vi "Init Module.vi"(7 "Create from class input? (F)":bool, 8 "error in (no error)":errorcluster, 9 "RSI Module in":refnum<class "RSI Module.lvclass">, 10 "Slot Settings":T1, 11 "Module Model":T2) -> (0 "error out":errorcluster, 3 "RSI Module out":refnum<class "RSI Module.lvclass">)   [LabVIEW 2017, in "Modules.lvlib"]
uses:
  Modules.lvlib
  RSI Module/Module Models.ctl
  RSI Module/Slot Settings.ctl
  RSI Module/RSI Module.lvclass
  RSI Module/Channels.ctl
  RSI Module/Channel Type.ctl
  9213/9213.lvclass
  C:/Users/nitest/Documents/niveristand-scan-engine-module-libraries/Source/RSI Module/RSI Module.lvclass
  9203/9203.lvclass
  9205/9205.lvclass
  9207/9207.lvclass
  9211/9211.lvclass
  9212/9212.lvclass
  9214/9214.lvclass
  9217/9217.lvclass
  9219/9219.lvclass
  9229/9229.lvclass
  9233/9233.lvclass
  9234/9234.lvclass
  9235/9235.lvclass
  9237/9237.lvclass
  9239/9239.lvclass
  9242/9242.lvclass
  9244/9244.lvclass
  9401/9401.lvclass
  9402/9402.lvclass
  9403/9403.lvclass
  9478/9478.lvclass
  SD Module/SD Module.lvclass
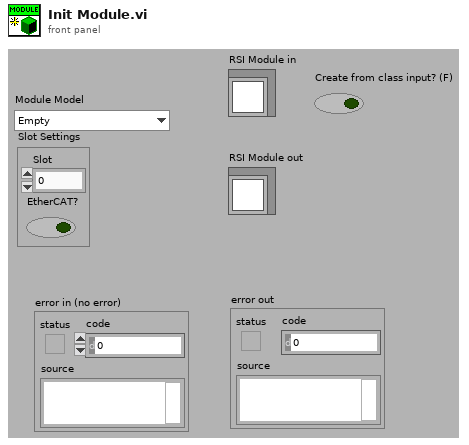
[diagram p1: front panel]
types:
  T1 = typedef "Modules.lvlib/RSI Module.lvclass/Slot Settings.ctl" = cluster{"Slot":u32, "EtherCAT?":bool}
  T2 = typedef "Modules.lvlib/RSI Module.lvclass/Module Models.ctl" = enum16{"Empty", "NI 9201", "NI 9203", "NI 9205", "NI 9206", "NI 9207", "NI 9208", "NI 9211", "NI 9212", "NI 9213", "NI 9214", "NI 9215", "NI 9217", "NI 9219", "NI 9220", "NI 9221", "NI 9222", "NI 9223", "NI 9224", "NI 9225", "NI 9227", "NI 9229", "NI 9233", "NI 9234", "NI 9235", "NI 9236", "NI 9237", "NI 9239", "NI 9242", "NI 9244", "NI 9263", "NI 9264", "NI 9265", "NI 9266", "NI 9269", "NI 9375", "NI 9401", "NI 9402", "NI 9403", "NI 9411", "NI 9421", "NI 9422", "NI 9423", "NI 9425", "NI 9426", "NI 9435", "NI 9437", "NI 9472", "NI 9474", "NI 9475", "NI 9476", "NI 9477", "NI 9478", "NI 9481", "NI 9482", "NI 9485"}
  T3 = typedef "Modules.lvlib/RSI Module.lvclass/Channels.ctl" = cluster{"# Input Channels":i32, "# Output Channels":i32, "Channel Type":T4, "Units":string}
  T4 = typedef "Modules.lvlib/RSI Module.lvclass/Channel Type.ctl" = enum16{"Analog", "Digital"}
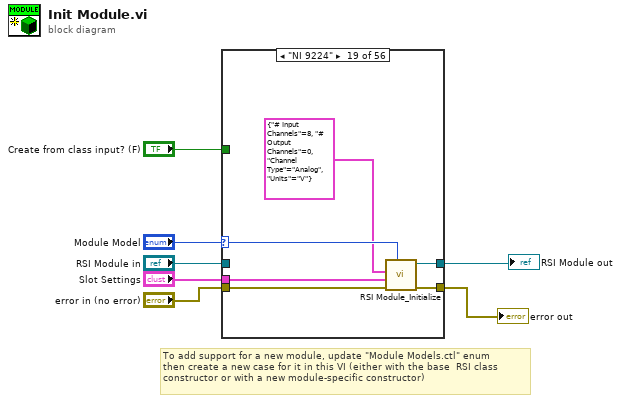
[diagram p0: block diagram]
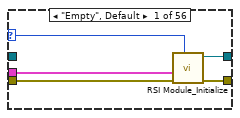
[diagram p2: hidden frame]
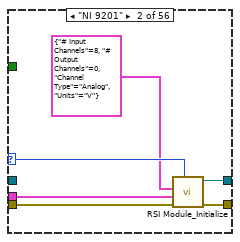
[diagram p3: hidden frame]
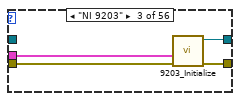
[diagram p4: hidden frame]
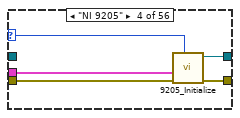
[diagram p5: hidden frame]
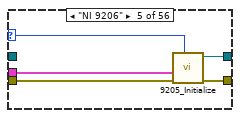
[diagram p6: hidden frame]
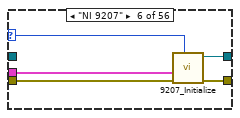
[diagram p7: hidden frame]
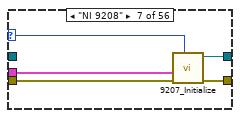
[diagram p8: hidden frame]
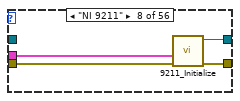
[diagram p9: hidden frame]
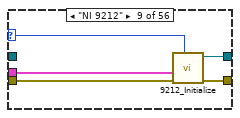
[diagram p10: hidden frame]
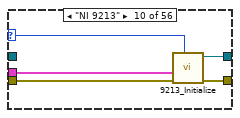
[diagram p11: hidden frame]
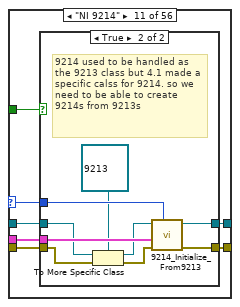
[diagram p12: hidden frame]
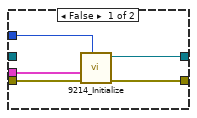
[diagram p13: hidden frame]
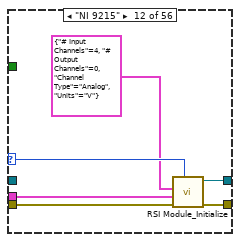
[diagram p14: hidden frame]
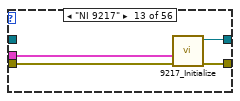
[diagram p15: hidden frame]
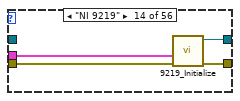
[diagram p16: hidden frame]
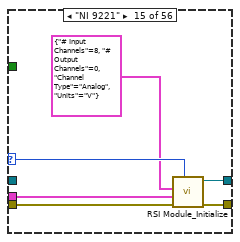
[diagram p17: hidden frame]
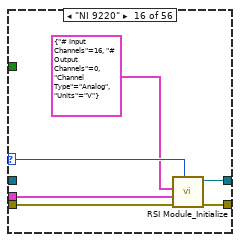
[diagram p18: hidden frame]
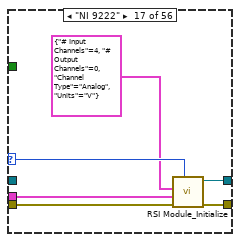
[diagram p19: hidden frame]
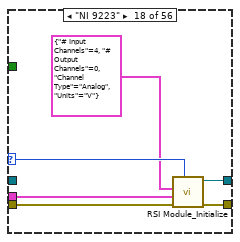
[diagram p20: hidden frame]
diagram:
  # "To add support for a new module, update \"Module Models.ctl\" enum\nthen create a new case for it in this VI (either with the base  RSI class\nconstructor or with a new module-specific constructor)"
  n1 = case shown="\"NI 9224\"" "Module Model" {
    selector: "Module Model" -> [w8 w18 _ w23 w29 w33 w38 _ w47 w52 w59 w83 _ _ w97 w103 w109 w115 w121 w127 w133 _ _ _ w146 w151 _ _ _ _ w177 w183 w189 w195 w201 w207 _ _ _ w226 w242 w260 w280 w301 w307 w310 w330 w348 w365 w386 w408 w414 _ w424 w430 w436]
    tunnel: [w11 w17 w19 w25 w31 w35 w40 w44 w50 w55 w62 w82 w87 w91 w96 w102 w108 w114 w120 w126 w132 w136 w140 w145 w150 w155 w157 w162 w164 w168 w176 w182 w188 w194 w200 w206 w211 w215 w219 w225 w244 w262 w282 w300 w306 w313 w332 w351 w370 w389 w407 w413 w417 w423 w429 w435] -> w3
    tunnel: [w12 w16 w22 w26 w32 w36 w41 w45 w51 w56 w63 w81 w86 w90 w95 w101 w107 w113 w119 w125 w131 w137 w141 w144 w147 w152 w156 w163 w167 w171 w175 w181 w187 w193 w199 w205 w210 w214 w218 w224 w243 w263 w277 w299 w305 w312 w331 w350 w369 w388 w406 w412 w418 w422 w428 w434] -> w6
    tunnel: "Slot Settings" -> [w9 w14 w20 w27 w28 w37 w42 w46 w48 w53 w60 w79 w85 w89 w93 w99 w105 w111 w117 w123 w129 w134 w139 w143 w148 w153 w158 w160 w165 w169 w173 w179 w185 w191 w197 w203 w209 w213 w217 w221 w240 w259 w279 w297 w303 w309 w328 w346 w367 w384 w404 w410 w415 w420 w426 w432]
    tunnel: "error in (no error)" -> [w10 w13 w21 w24 w30 w34 w39 w43 w49 w54 w61 w78 w84 w88 w92 w98 w104 w110 w116 w122 w128 w135 w138 w142 w149 w154 w159 w161 w166 w170 w172 w178 w184 w190 w196 w202 w208 w212 w216 w222 w241 w258 w278 w296 w302 w308 w329 w347 w368 w385 w403 w409 w416 w419 w425 w431]
    tunnel: "Create from class input? (F)" -> [_ _ _ _ _ _ _ _ _ _ w58 _ _ _ _ _ _ _ _ _ _ _ _ _ _ _ _ _ _ _ _ _ _ _ _ _ _ _ _ _ _ _ _ _ _ _ _ _ _ _ _ _ _ _ _ _]
    tunnel: "RSI Module in" -> [_ _ _ _ _ _ _ _ _ _ w57 _ _ _ _ _ _ _ _ _ _ _ _ _ _ _ _ _ _ _ _ _ _ _ _ _ _ _ _ _ _ _ _ _ _ _ _ _ _ _ _ _ _ _ _ _]
    frame "Empty", Default {
      n2 = call "RSI Module_Initialize.vi"("Module Model"=w8, "error in (no error)"=w10, "Slot Settings"=w9) -> ("error out"=w12:errorcluster, "RSI Module out"=w11:refnum<class "RSI Module.lvclass">)  [unwired: 7 in]
    }
    frame "NI 9201" {
      n3 = call "RSI Module_Initialize.vi"("Module Model"=w18, "error in (no error)"=w13, "Slot Settings"=w14, "Channels"=T3 {"# Input Channels"=8, "# Output Channels"=0, "Channel Type"=enum."Analog", "Units"="V"}) -> ("error out"=w16:errorcluster, "RSI Module out"=w17:refnum<class "RSI Module.lvclass">)  [unwired: 6 in]
    }
    frame "NI 9203" {
      n4 = call "9203_Initialize.vi"("error in (no error)"=w21, "Slot Settings"=w20) -> ("error out"=w22:errorcluster, "9203 out"=w19:refnum<class "9203.lvclass">)  [unwired: 8 in]
    }
    frame "NI 9205" {
      n5 = call "9205_Initialize.vi"("Module Model"=w23, "error in (no error)"=w24, "Slot Settings"=w27) -> ("error out"=w26:errorcluster, "9205 out"=w25:refnum<class "9205.lvclass">)  [unwired: 7 in]
    }
    frame "NI 9206" {
      n6 = call "9205_Initialize.vi"("Module Model"=w29, "error in (no error)"=w30, "Slot Settings"=w28) -> ("error out"=w32:errorcluster, "9205 out"=w31:refnum<class "9205.lvclass">)  [unwired: 7 in]
    }
    frame "NI 9207" {
      n7 = call "9207_Initialize.vi"("Module Model"=w33, "error in (no error)"=w34, "Slot Settings"=w37) -> ("error out"=w36:errorcluster, "9207 out"=w35:refnum<class "9207.lvclass">)  [unwired: 7 in]
    }
    frame "NI 9208" {
      n8 = call "9207_Initialize.vi"("Module Model"=w38, "error in (no error)"=w39, "Slot Settings"=w42) -> ("error out"=w41:errorcluster, "9207 out"=w40:refnum<class "9207.lvclass">)  [unwired: 7 in]
    }
    frame "NI 9211" {
      n9 = call "9211_Initialize.vi"("error in (no error)"=w43, "Slot Settings"=w46) -> ("error out"=w45:errorcluster, "9211 out"=w44:refnum<class "9211.lvclass">)  [unwired: 8 in]
    }
    frame "NI 9212" {
      n10 = call "9212_Initialize.vi"("Module Model"=w47, "error in (no error)"=w49, "Slot Settings"=w48) -> ("error out"=w51:errorcluster, "9213 out"=w50:refnum<class "9212.lvclass">)  [unwired: 7 in]
    }
    frame "NI 9213" {
      n11 = call "9213_Initialize.vi"("Module Model"=w52, "error in (no error)"=w54, "Slot Settings"=w53) -> ("error out"=w56:errorcluster, "9213 out"=w55:refnum<class "9213.lvclass">)  [unwired: 7 in]
    }
    frame "NI 9214" {
      n12 = case shown="True" w58 {
        tunnel: [w68 w77] -> w63
        tunnel: [w67 w76] -> w62
        tunnel: w61 -> [w66 w73]
        tunnel: w60 -> [w65 w75]
        tunnel: w59 -> [w64 w74]
        tunnel: w57 -> [_ w72]
        frame False {
          n13 = call "9214_Initialize.vi"("Module Model"=w64, "error in (no error)"=w66, "Slot Settings"=w65) -> ("error out"=w68:errorcluster, "9214 out"=w67:refnum<class "9214.lvclass">)  [unwired: 7 in]
        }
        frame True {
          # "9214 used to be handled as the 9213 class but 4.1 made a specific calss for 9214. so we need to be able to create 9214s from 9213s"
          n14 = To More Specific Class(target class=refnum<class "9213.lvclass"> refnum ("Modules.lvlib:9213.lvclass"), reference=w72, error in=w73) -> (specific class reference=w70:refnum<class "9213.lvclass">, error out=w69:errorcluster)
          n15 = call "9214_Initialize_From9213.vi"("Module Model"=w74, "error in (no error)"=w69, "Slot Settings"=w75, "9213 in"=w70) -> ("error out"=w77:errorcluster, "9214 out"=w76:refnum<class "9214.lvclass">)  [unwired: 6 in]
        }
      }
    }
    frame "NI 9215" {
      n16 = call "RSI Module_Initialize.vi"("Module Model"=w83, "error in (no error)"=w78, "Slot Settings"=w79, "Channels"=T3 {"# Input Channels"=4, "# Output Channels"=0, "Channel Type"=enum."Analog", "Units"="V"}) -> ("error out"=w81:errorcluster, "RSI Module out"=w82:refnum<class "RSI Module.lvclass">)  [unwired: 6 in]
    }
    frame "NI 9217" {
      n17 = call "9217_Initialize.vi"("error in (no error)"=w84, "Slot Settings"=w85) -> ("error out"=w86:errorcluster, "9217 out"=w87:refnum<class "9217.lvclass">)  [unwired: 8 in]
    }
    frame "NI 9219" {
      n18 = call "9219_Initialize.vi"("error in (no error)"=w88, "Slot Settings"=w89) -> ("error out"=w90:errorcluster, "9219 out"=w91:refnum<class "9219.lvclass">)  [unwired: 8 in]
    }
    frame "NI 9221" {
      n19 = call "RSI Module_Initialize.vi"("Module Model"=w97, "error in (no error)"=w92, "Slot Settings"=w93, "Channels"=T3 {"# Input Channels"=8, "# Output Channels"=0, "Channel Type"=enum."Analog", "Units"="V"}) -> ("error out"=w95:errorcluster, "RSI Module out"=w96:refnum<class "RSI Module.lvclass">)  [unwired: 6 in]
    }
    frame "NI 9220" {
      n20 = call "RSI Module_Initialize.vi"("Module Model"=w103, "error in (no error)"=w98, "Slot Settings"=w99, "Channels"=T3 {"# Input Channels"=16, "# Output Channels"=0, "Channel Type"=enum."Analog", "Units"="V"}) -> ("error out"=w101:errorcluster, "RSI Module out"=w102:refnum<class "RSI Module.lvclass">)  [unwired: 6 in]
    }
    frame "NI 9222" {
      n21 = call "RSI Module_Initialize.vi"("Module Model"=w109, "error in (no error)"=w104, "Slot Settings"=w105, "Channels"=T3 {"# Input Channels"=4, "# Output Channels"=0, "Channel Type"=enum."Analog", "Units"="V"}) -> ("error out"=w107:errorcluster, "RSI Module out"=w108:refnum<class "RSI Module.lvclass">)  [unwired: 6 in]
    }
    frame "NI 9223" {
      n22 = call "RSI Module_Initialize.vi"("Module Model"=w115, "error in (no error)"=w110, "Slot Settings"=w111, "Channels"=T3 {"# Input Channels"=4, "# Output Channels"=0, "Channel Type"=enum."Analog", "Units"="V"}) -> ("error out"=w113:errorcluster, "RSI Module out"=w114:refnum<class "RSI Module.lvclass">)  [unwired: 6 in]
    }
    frame "NI 9224" {
      n23 = call "RSI Module_Initialize.vi"("Module Model"=w121, "error in (no error)"=w116, "Slot Settings"=w117, "Channels"=T3 {"# Input Channels"=8, "# Output Channels"=0, "Channel Type"=enum."Analog", "Units"="V"}) -> ("error out"=w119:errorcluster, "RSI Module out"=w120:refnum<class "RSI Module.lvclass">)  [unwired: 6 in]
    }
    frame "NI 9225" {
      n24 = call "RSI Module_Initialize.vi"("Module Model"=w127, "error in (no error)"=w122, "Slot Settings"=w123, "Channels"=T3 {"# Input Channels"=3, "# Output Channels"=0, "Channel Type"=enum."Analog", "Units"="Vrms"}) -> ("error out"=w125:errorcluster, "RSI Module out"=w126:refnum<class "RSI Module.lvclass">)  [unwired: 6 in]
    }
    frame "NI 9227" {
      n25 = call "RSI Module_Initialize.vi"("Module Model"=w133, "error in (no error)"=w128, "Slot Settings"=w129, "Channels"=T3 {"# Input Channels"=4, "# Output Channels"=0, "Channel Type"=enum."Analog", "Units"="Arms"}) -> ("error out"=w131:errorcluster, "RSI Module out"=w132:refnum<class "RSI Module.lvclass">)  [unwired: 6 in]
    }
    frame "NI 9229" {
      n26 = call "9229_Initialize.vi"("error in (no error)"=w135, "Slot Settings"=w134) -> ("error out"=w137:errorcluster, "9229 out"=w136:refnum<class "9229.lvclass">)  [unwired: 8 in]
    }
    frame "NI 9233" {
      n27 = call "9233_Initialize.vi"("error in (no error)"=w138, "Slot Settings"=w139) -> ("error out"=w141:errorcluster, "9233 out"=w140:refnum<class "9233.lvclass">)  [unwired: 8 in]
    }
    frame "NI 9234" {
      n28 = call "9234_Initialize.vi"("error in (no error)"=w142, "Slot Settings"=w143) -> ("error out"=w144:errorcluster, "9234 out"=w145:refnum<class "9234.lvclass">)  [unwired: 8 in]
    }
    frame "NI 9235" {
      n29 = call "9235_Initialize.vi"("Module Model"=w146, "error in (no error)"=w149, "Slot Settings"=w148) -> ("error out"=w147:errorcluster, "9235 out"=w150:refnum<class "9235.lvclass">)  [unwired: 7 in]
    }
    frame "NI 9236" {
      n30 = call "9235_Initialize.vi"("Module Model"=w151, "error in (no error)"=w154, "Slot Settings"=w153) -> ("error out"=w152:errorcluster, "9235 out"=w155:refnum<class "9235.lvclass">)  [unwired: 7 in]
    }
    frame "NI 9237" {
      n31 = call "9237_Initialize.vi"("error in (no error)"=w159, "Slot Settings"=w158) -> ("error out"=w156:errorcluster, "9237 out"=w157:refnum<class "9237.lvclass">)  [unwired: 8 in]
    }
    frame "NI 9239" {
      n32 = call "9239_Initialize.vi"("error in (no error)"=w161, "Slot Settings"=w160) -> ("error out"=w163:errorcluster, "9239 out"=w162:refnum<class "9239.lvclass">)  [unwired: 8 in]
    }
    frame "NI 9242" {
      n33 = call "9242_Initialize.vi"("error in (no error)"=w166, "Slot Settings"=w165) -> ("error out"=w167:errorcluster, "Modules.lvlib:9242.lvclass"=w164:refnum<class "9242.lvclass">)  [unwired: 8 in]
    }
    frame "NI 9244" {
      n34 = call "9244_Initialize.vi"("error in (no error)"=w170, "Slot Settings"=w169) -> ("error out"=w171:errorcluster, "Modules.lvlib:9244.lvclass"=w168:refnum<class "9244.lvclass">)  [unwired: 8 in]
    }
    frame "NI 9263" {
      n35 = call "RSI Module_Initialize.vi"("Module Model"=w177, "error in (no error)"=w172, "Slot Settings"=w173, "Channels"=T3 {"# Input Channels"=0, "# Output Channels"=4, "Channel Type"=enum."Analog", "Units"="V"}) -> ("error out"=w175:errorcluster, "RSI Module out"=w176:refnum<class "RSI Module.lvclass">)  [unwired: 6 in]
    }
    frame "NI 9264" {
      n36 = call "RSI Module_Initialize.vi"("Module Model"=w183, "error in (no error)"=w178, "Slot Settings"=w179, "Channels"=T3 {"# Input Channels"=0, "# Output Channels"=16, "Channel Type"=enum."Analog", "Units"="V"}) -> ("error out"=w181:errorcluster, "RSI Module out"=w182:refnum<class "RSI Module.lvclass">)  [unwired: 6 in]
    }
    frame "NI 9265" {
      n37 = call "RSI Module_Initialize.vi"("Module Model"=w189, "error in (no error)"=w184, "Slot Settings"=w185, "Channels"=T3 {"# Input Channels"=0, "# Output Channels"=4, "Channel Type"=enum."Analog", "Units"="A"}) -> ("error out"=w187:errorcluster, "RSI Module out"=w188:refnum<class "RSI Module.lvclass">)  [unwired: 6 in]
    }
    frame "NI 9266" {
      n38 = call "RSI Module_Initialize.vi"("Module Model"=w195, "error in (no error)"=w190, "Slot Settings"=w191, "Channels"=T3 {"# Input Channels"=0, "# Output Channels"=8, "Channel Type"=enum."Analog", "Units"="A"}) -> ("error out"=w193:errorcluster, "RSI Module out"=w194:refnum<class "RSI Module.lvclass">)  [unwired: 6 in]
    }
    frame "NI 9269" {
      n39 = call "RSI Module_Initialize.vi"("Module Model"=w201, "error in (no error)"=w196, "Slot Settings"=w197, "Channels"=T3 {"# Input Channels"=0, "# Output Channels"=4, "Channel Type"=enum."Analog", "Units"="V"}) -> ("error out"=w199:errorcluster, "RSI Module out"=w200:refnum<class "RSI Module.lvclass">)  [unwired: 6 in]
    }
    frame "NI 9375" {
      n40 = call "RSI Module_Initialize.vi"("Module Model"=w207, "error in (no error)"=w202, "Slot Settings"=w203, "Channels"=T3 {"# Input Channels"=16, "# Output Channels"=16, "Channel Type"=enum."Digital", "Units"=""}) -> ("error out"=w205:errorcluster, "RSI Module out"=w206:refnum<class "RSI Module.lvclass">)  [unwired: 6 in]
    }
    frame "NI 9401" {
      n41 = call "9401_Initialize.vi"("error in (no error)"=w208, "Slot Settings"=w209) -> ("error out"=w210:errorcluster, "9401 out"=w211:refnum<class "9401.lvclass">)  [unwired: 8 in]
    }
    frame "NI 9402" {
      n42 = call "9402_Initialize.vi"("error in (no error)"=w212, "Slot Settings"=w213) -> ("error out"=w214:errorcluster, "9402 out"=w215:refnum<class "9402.lvclass">)  [unwired: 8 in]
    }
    frame "NI 9403" {
      n43 = call "9403_Initialize.vi"("error in (no error)"=w216, "Slot Settings"=w217) -> ("error out"=w218:errorcluster, "9403 out"=w219:refnum<class "9403.lvclass">)  [unwired: 8 in]
    }
    frame "NI 9411" {
      n44 = Unbundle By Name(w221) -> ("EtherCAT?"=w220:bool)
      n45 = case shown="True" w220 {
        tunnel: w226 -> [w232 w235]
        tunnel: [w231 w236] -> w225
        tunnel: [w230 w237] -> w224
        tunnel: T3 {"# Input Channels"=6, "# Output Channels"=0, "Channel Type"=enum."Digital", "Units"=""} ("Channels") -> [w229 w234]
        tunnel: w222 -> [w228 w238]
        tunnel: w221 -> [w227 w233]
        frame False {
          n46 = call "SD Module_Initialize.vi"("Module Model"=w232, "error in (no error)"=w228, "Slot Settings"=w227, "Channels"=w229) -> ("error out"=w230:errorcluster, "SD Module out"=w231:refnum<class "SD Module.lvclass">)  [unwired: 6 in]
        }
        frame True {
          n47 = call "RSI Module_Initialize.vi"("Module Model"=w235, "error in (no error)"=w238, "Slot Settings"=w233, "Channels"=w234) -> ("error out"=w237:errorcluster, "RSI Module out"=w236:refnum<class "RSI Module.lvclass">)  [unwired: 6 in]
        }
      }
    }
    frame "NI 9421" {
      n48 = Unbundle By Name(w240) -> ("EtherCAT?"=w245:bool)
      n49 = case shown="True" w245 {
        tunnel: w242 -> [w251 w254]
        tunnel: [w250 w255] -> w244
        tunnel: [w249 w256] -> w243
        tunnel: T3 {"# Input Channels"=8, "# Output Channels"=0, "Channel Type"=enum."Digital", "Units"=""} ("Channels") -> [w248 w253]
        tunnel: w241 -> [w247 w257]
        tunnel: w240 -> [w246 w252]
        frame False {
          n50 = call "SD Module_Initialize.vi"("Module Model"=w251, "error in (no error)"=w247, "Slot Settings"=w246, "Channels"=w248) -> ("error out"=w249:errorcluster, "SD Module out"=w250:refnum<class "SD Module.lvclass">)  [unwired: 6 in]
        }
        frame True {
          n51 = call "RSI Module_Initialize.vi"("Module Model"=w254, "error in (no error)"=w257, "Slot Settings"=w252, "Channels"=w253) -> ("error out"=w256:errorcluster, "RSI Module out"=w255:refnum<class "RSI Module.lvclass">)  [unwired: 6 in]
        }
      }
    }
    frame "NI 9422" {
      n52 = Unbundle By Name(w259) -> ("EtherCAT?"=w264:bool)
      n53 = case shown="True" w264 {
        tunnel: w260 -> [w270 w273]
        tunnel: [w269 w274] -> w262
        tunnel: [w268 w275] -> w263
        tunnel: T3 {"# Input Channels"=8, "# Output Channels"=0, "Channel Type"=enum."Digital", "Units"=""} ("Channels") -> [w267 w272]
        tunnel: w258 -> [w266 w276]
        tunnel: w259 -> [w265 w271]
        frame False {
          n54 = call "SD Module_Initialize.vi"("Module Model"=w270, "error in (no error)"=w266, "Slot Settings"=w265, "Channels"=w267) -> ("error out"=w268:errorcluster, "SD Module out"=w269:refnum<class "SD Module.lvclass">)  [unwired: 6 in]
        }
        frame True {
          n55 = call "RSI Module_Initialize.vi"("Module Model"=w273, "error in (no error)"=w276, "Slot Settings"=w271, "Channels"=w272) -> ("error out"=w275:errorcluster, "RSI Module out"=w274:refnum<class "RSI Module.lvclass">)  [unwired: 6 in]
        }
      }
    }
    frame "NI 9423" {
      n56 = Unbundle By Name(w279) -> ("EtherCAT?"=w283:bool)
      n57 = case shown="False" w283 {
        tunnel: w280 -> [w289 w292]
        tunnel: [w288 w293] -> w282
        tunnel: [w287 w294] -> w277
        tunnel: T3 {"# Input Channels"=8, "# Output Channels"=0, "Channel Type"=enum."Digital", "Units"=""} ("Channels") -> [w286 w291]
        tunnel: w278 -> [w285 w295]
        tunnel: w279 -> [w284 w290]
        frame False {
          n58 = call "SD Module_Initialize.vi"("Module Model"=w289, "error in (no error)"=w285, "Slot Settings"=w284, "Channels"=w286) -> ("error out"=w287:errorcluster, "SD Module out"=w288:refnum<class "SD Module.lvclass">)  [unwired: 6 in]
        }
        frame True {
          n59 = call "RSI Module_Initialize.vi"("Module Model"=w292, "error in (no error)"=w295, "Slot Settings"=w290, "Channels"=w291) -> ("error out"=w294:errorcluster, "RSI Module out"=w293:refnum<class "RSI Module.lvclass">)  [unwired: 6 in]
        }
      }
    }
    frame "NI 9425" {
      n60 = call "RSI Module_Initialize.vi"("Module Model"=w301, "error in (no error)"=w296, "Slot Settings"=w297, "Channels"=T3 {"# Input Channels"=32, "# Output Channels"=0, "Channel Type"=enum."Digital", "Units"=""}) -> ("error out"=w299:errorcluster, "RSI Module out"=w300:refnum<class "RSI Module.lvclass">)  [unwired: 6 in]
    }
    frame "NI 9426" {
      n61 = call "RSI Module_Initialize.vi"("Module Model"=w307, "error in (no error)"=w302, "Slot Settings"=w303, "Channels"=T3 {"# Input Channels"=32, "# Output Channels"=0, "Channel Type"=enum."Digital", "Units"=""}) -> ("error out"=w305:errorcluster, "RSI Module out"=w306:refnum<class "RSI Module.lvclass">)  [unwired: 6 in]
    }
    frame "NI 9435" {
      n62 = Unbundle By Name(w309) -> ("EtherCAT?"=w314:bool)
      n63 = case shown="True" w314 {
        tunnel: w310 -> [w320 w323]
        tunnel: [w319 w324] -> w313
        tunnel: [w318 w325] -> w312
        tunnel: T3 {"# Input Channels"=4, "# Output Channels"=0, "Channel Type"=enum."Digital", "Units"=""} ("Channels") -> [w317 w322]
        tunnel: w308 -> [w316 w326]
        tunnel: w309 -> [w315 w321]
        frame False {
          n64 = call "SD Module_Initialize.vi"("Module Model"=w320, "error in (no error)"=w316, "Slot Settings"=w315, "Channels"=w317) -> ("error out"=w318:errorcluster, "SD Module out"=w319:refnum<class "SD Module.lvclass">)  [unwired: 6 in]
        }
        frame True {
          n65 = call "RSI Module_Initialize.vi"("Module Model"=w323, "error in (no error)"=w326, "Slot Settings"=w321, "Channels"=w322) -> ("error out"=w325:errorcluster, "RSI Module out"=w324:refnum<class "RSI Module.lvclass">)  [unwired: 6 in]
        }
      }
    }
    frame "NI 9437" {
      n66 = Unbundle By Name(w328) -> ("EtherCAT?"=w333:bool)
      n67 = case shown="False" w333 {
        tunnel: w330 -> [w339 w342]
        tunnel: [w338 w343] -> w332
        tunnel: [w337 w344] -> w331
        tunnel: T3 {"# Input Channels"=8, "# Output Channels"=0, "Channel Type"=enum."Digital", "Units"=""} ("Channels") -> [w336 w341]
        tunnel: w329 -> [w335 w345]
        tunnel: w328 -> [w334 w340]
        frame False {
          n68 = call "SD Module_Initialize.vi"("Module Model"=w339, "error in (no error)"=w335, "Slot Settings"=w334, "Channels"=w336) -> ("error out"=w337:errorcluster, "SD Module out"=w338:refnum<class "SD Module.lvclass">)  [unwired: 6 in]
        }
        frame True {
          n69 = call "RSI Module_Initialize.vi"("Module Model"=w342, "error in (no error)"=w345, "Slot Settings"=w340, "Channels"=w341) -> ("error out"=w344:errorcluster, "RSI Module out"=w343:refnum<class "RSI Module.lvclass">)  [unwired: 6 in]
        }
      }
    }
    frame "NI 9472" {
      n70 = Unbundle By Name(w346) -> ("EtherCAT?"=w352:bool)
      n71 = case shown="True" w352 {
        tunnel: w348 -> [w358 w361]
        tunnel: [w357 w362] -> w351
        tunnel: [w356 w363] -> w350
        tunnel: T3 {"# Input Channels"=0, "# Output Channels"=8, "Channel Type"=enum."Digital", "Units"=""} ("Channels") -> [w355 w360]
        tunnel: w347 -> [w354 w364]
        tunnel: w346 -> [w353 w359]
        frame False {
          n72 = call "SD Module_Initialize.vi"("Module Model"=w358, "error in (no error)"=w354, "Slot Settings"=w353, "Channels"=w355) -> ("error out"=w356:errorcluster, "SD Module out"=w357:refnum<class "SD Module.lvclass">)  [unwired: 6 in]
        }
        frame True {
          n73 = call "RSI Module_Initialize.vi"("Module Model"=w361, "error in (no error)"=w364, "Slot Settings"=w359, "Channels"=w360) -> ("error out"=w363:errorcluster, "RSI Module out"=w362:refnum<class "RSI Module.lvclass">)  [unwired: 6 in]
        }
      }
    }
    frame "NI 9474" {
      n74 = Unbundle By Name(w367) -> ("EtherCAT?"=w371:bool)
      n75 = case shown="False" w371 {
        tunnel: w365 -> [w377 w380]
        tunnel: [w376 w381] -> w370
        tunnel: [w375 w382] -> w369
        tunnel: T3 {"# Input Channels"=0, "# Output Channels"=8, "Channel Type"=enum."Digital", "Units"=""} ("Channels") -> [w374 w379]
        tunnel: w368 -> [w373 w383]
        tunnel: w367 -> [w372 w378]
        frame False {
          n76 = call "SD Module_Initialize.vi"("Module Model"=w377, "error in (no error)"=w373, "Slot Settings"=w372, "Channels"=w374) -> ("error out"=w375:errorcluster, "SD Module out"=w376:refnum<class "SD Module.lvclass">)  [unwired: 6 in]
        }
        frame True {
          n77 = call "RSI Module_Initialize.vi"("Module Model"=w380, "error in (no error)"=w383, "Slot Settings"=w378, "Channels"=w379) -> ("error out"=w382:errorcluster, "RSI Module out"=w381:refnum<class "RSI Module.lvclass">)  [unwired: 6 in]
        }
      }
    }
    frame "NI 9475" {
      n78 = Unbundle By Name(w384) -> ("EtherCAT?"=w390:bool)
      n79 = case shown="True" w390 {
        tunnel: w386 -> [w396 w399]
        tunnel: [w395 w400] -> w389
        tunnel: [w394 w401] -> w388
        tunnel: T3 {"# Input Channels"=0, "# Output Channels"=8, "Channel Type"=enum."Digital", "Units"=""} ("Channels") -> [w393 w398]
        tunnel: w385 -> [w392 w402]
        tunnel: w384 -> [w391 w397]
        frame False {
          n80 = call "SD Module_Initialize.vi"("Module Model"=w396, "error in (no error)"=w392, "Slot Settings"=w391, "Channels"=w393) -> ("error out"=w394:errorcluster, "SD Module out"=w395:refnum<class "SD Module.lvclass">)  [unwired: 6 in]
        }
        frame True {
          n81 = call "RSI Module_Initialize.vi"("Module Model"=w399, "error in (no error)"=w402, "Slot Settings"=w397, "Channels"=w398) -> ("error out"=w401:errorcluster, "RSI Module out"=w400:refnum<class "RSI Module.lvclass">)  [unwired: 6 in]
        }
      }
    }
    frame "NI 9476" {
      n82 = call "RSI Module_Initialize.vi"("Module Model"=w408, "error in (no error)"=w403, "Slot Settings"=w404, "Channels"=T3 {"# Input Channels"=0, "# Output Channels"=32, "Channel Type"=enum."Digital", "Units"=""}) -> ("error out"=w406:errorcluster, "RSI Module out"=w407:refnum<class "RSI Module.lvclass">)  [unwired: 6 in]
    }
    frame "NI 9477" {
      n83 = call "RSI Module_Initialize.vi"("Module Model"=w414, "error in (no error)"=w409, "Slot Settings"=w410, "Channels"=T3 {"# Input Channels"=0, "# Output Channels"=32, "Channel Type"=enum."Digital", "Units"=""}) -> ("error out"=w412:errorcluster, "RSI Module out"=w413:refnum<class "RSI Module.lvclass">)  [unwired: 6 in]
    }
    frame "NI 9478" {
      n84 = call "9478_Initialize.vi"("error in (no error)"=w416, "Slot Settings"=w415) -> ("error out"=w418:errorcluster, "9478 out"=w417:refnum<class "9478.lvclass">)  [unwired: 8 in]
    }
    frame "NI 9481" {
      n85 = call "RSI Module_Initialize.vi"("Module Model"=w424, "error in (no error)"=w419, "Slot Settings"=w420, "Channels"=T3 {"# Input Channels"=0, "# Output Channels"=4, "Channel Type"=enum."Digital", "Units"=""}) -> ("error out"=w422:errorcluster, "RSI Module out"=w423:refnum<class "RSI Module.lvclass">)  [unwired: 6 in]
    }
    frame "NI 9482" {
      n86 = call "RSI Module_Initialize.vi"("Module Model"=w430, "error in (no error)"=w425, "Slot Settings"=w426, "Channels"=T3 {"# Input Channels"=0, "# Output Channels"=4, "Channel Type"=enum."Digital", "Units"=""}) -> ("error out"=w428:errorcluster, "RSI Module out"=w429:refnum<class "RSI Module.lvclass">)  [unwired: 6 in]
    }
    frame "NI 9485" {
      n87 = call "RSI Module_Initialize.vi"("Module Model"=w436, "error in (no error)"=w431, "Slot Settings"=w432, "Channels"=T3 {"# Input Channels"=0, "# Output Channels"=8, "Channel Type"=enum."Digital", "Units"=""}) -> ("error out"=w434:errorcluster, "RSI Module out"=w435:refnum<class "RSI Module.lvclass">)  [unwired: 6 in]
    }
  }
  "error out" <- w6
  "RSI Module out" <- w3
